vi "Hitrap_DiagnosticBoxGUI.set value.vi"(0 "i ref in":refnum<vi>, 1 "CallType":enum16{"simple", "synchronous", "asynchronous"}(ring)=enum."synchronous", 2 "Data Discriptor":string, 3 "Selector":string, 4 "Data":T1, 5 "error in (no error)":errorcluster) -> (19 "error out":errorcluster)   [LabVIEW 2014, in "Hitrap_DiagnosticBoxGUI.lvlib"]
doc: "calls the ProcCases of the DiagnosticBox"
uses:
  Hitrap_DiagnosticBoxGUI.lvlib
  CS_Core/CSSystem/CoreDefs/CoreDefs.call_type.ctl
  CS_Core/BaseProcess/BaseProcess.descriptor string definition.ctl
  CS_Core/CSSystem/CoreDefs/CoreDefs.rawDataType.ctl
  CS_Core/BaseProcess/BaseProcess.lvlib
  CS_Core/GUIs/GOGUserGUIs/DeviceBaseGUI/DeviceBaseGUI.lvlib
panel:
  out "call cluster out":T2={"Object"="", "Selector"="", "CallType"=enum."synchronous", "Async Object"="", "Async Selector"="", "Data Descriptor"="", "Data"=[], "Error #"=0, "Expire"=0}
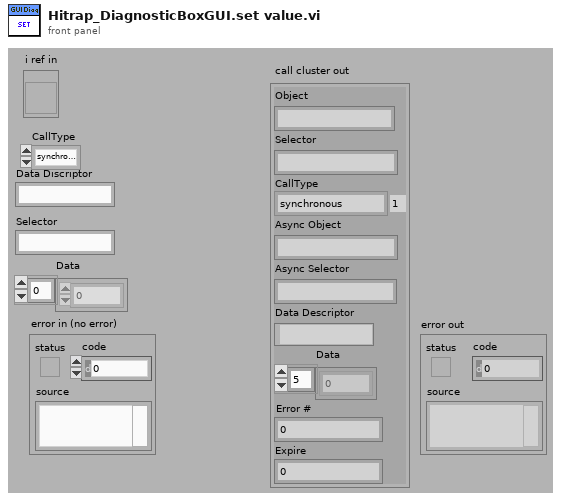
[diagram p1: front panel]
types:
  T1 = typedef "CoreDefs.rawDataType.ctl" = i8[]
  T2 = typedef "CoreDefs.call_type.ctl" = cluster{"Object":string, "Selector":string, "CallType":enum16{"simple", "synchronous", "asynchronous"}, "Async Object":string, "Async Selector":string, "Data Descriptor":T3, "Data":T1, "Error #":i32, "Expire":u32}
  T3 = typedef "BaseProcess.lvlib/BaseProcess.descriptor string definition.ctl" = string
  T4 = typedef "DeviceBaseGUI.lvlib/DeviceBaseGUI.i attribute.ctl" = cluster{"GOGFrontPanel.i attribute":T5}
  T5 = typedef "GOGFrontPanel.lvlib/GOGFrontPanel.i attribute.ctl" = cluster{"GOGObject":string, "Object":string, "Method":string, "Descriptor":T3, "Input Descriptor":string, "Output Descriptor":string, "inputNames":string[], "outputNames":string[], "Values":cluster{"descriptor":string, "value":string}[]}
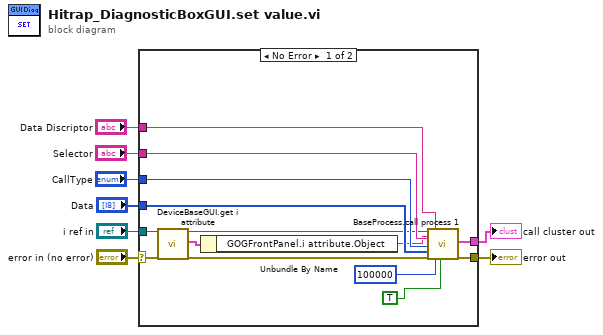
[diagram p0: block diagram]
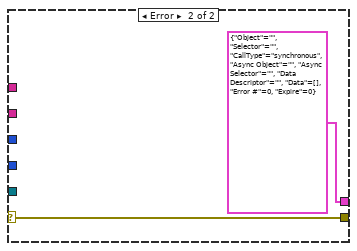
[diagram p2: hidden frame]
diagram:
  n1 = case shown="No Error" "error in (no error)" {
    selector: "error in (no error)" -> [w12 w24]
    tunnel: [w22 T2 {"Object"="", "Selector"="", "CallType"=enum."synchronous", "Async Object"="", "Async Selector"="", "Data Descriptor"="", "Data"=[], "Error #"=0, "Expire"=0} ("call cluster out")] -> w8
    tunnel: "i ref in" -> [w14 _]
    tunnel: "Data" -> [w21 _]
    tunnel: "Selector" -> [w20 _]
    tunnel: "Data Discriptor" -> [w19 _]
    tunnel: [w18 w24] -> w2
    tunnel: "CallType" -> [w15 _]
    frame No Error {
      n2 = call "DeviceBaseGUI.get i attribute.vi"("i ref in"=w14, "error in (no error)"=w12) -> ("i ref out"=w13:refnum<vi>, "i attribute"=w10:T4, "error out"=w11:errorcluster)  [unwired: 15 in]
      n3 = Unbundle By Name(w10) -> ("GOGFrontPanel.i attribute.Object"=w9:string)
      n4 = call "BaseProcess.call process 1.vi"("i ref in"=w13, "Object"=w9, "Selector"=w20, "CallType"=w15, "Data"=w21, "error in (no error)"=w11, "Data Descriptor"=w19, "timeout (ms)"=100000, "expire"=TRUE) -> ("call cluster out"=w22:T2, "error out"=w18:errorcluster)  [unwired: 8 in, 1 out]
    }
    frame Error {
    }
  }
  "call cluster out" <- w8
  "error out" <- w2
